vi "Read Multiple Voltage Measurements.vi"(8 "error in (no error)":errorcluster, 10 "Multiple Voltage Measurement Type (0:DC)":u16(ring) items=["Voltage", "Voltage Harmonic Amplitude", "Voltage Harmonic Phase"], 11 "VISA resource name":refnum<visa-resource-name>) -> (0 "error out":errorcluster, 2 "Voltage Measurements":sgl[](array[numeric]), 3 "VISA resource name out":refnum<visa-resource-name>)   [LabVIEW 2013, in "California Instruments iX Series.lvlib"]
doc: "Reads the multiple voltage measurements based on the user selectable measurement type."
uses:
  California Instruments iX Series.lvlib
panel:
  out "size(s)":i32
  out "Serial Settings:Number of Bytes at Serial Port":u32
  out "return count":u32
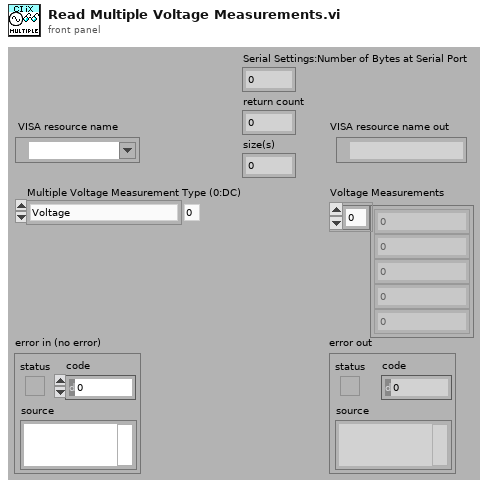
[diagram p1: front panel]
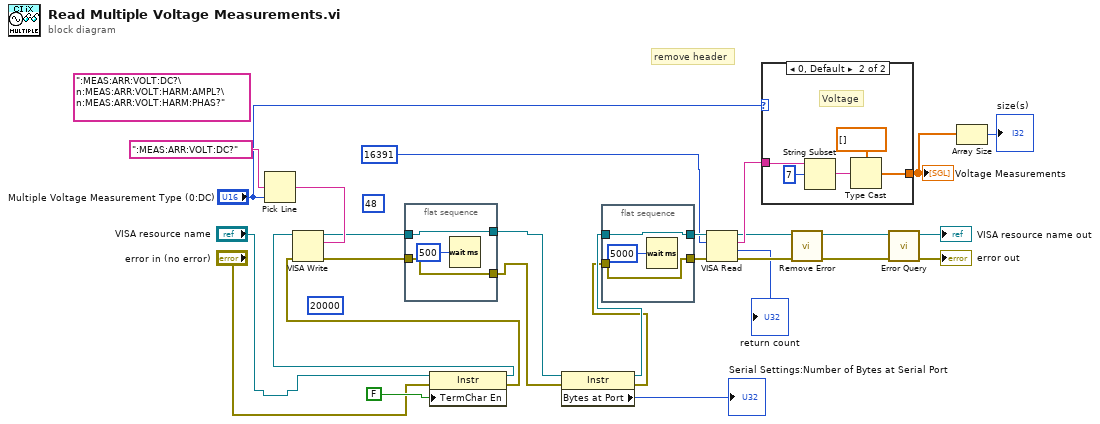
[diagram p0: block diagram]
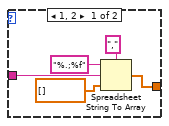
[diagram p2: hidden frame]
diagram:
  (unwired) u16 48 ("mask (16)")
  (unwired) u32 20000 ("size (4096)")
  (unwired) ":MEAS:ARR:VOLT:DC?\n:MEAS:ARR:VOLT:HARM:AMPL?\n:MEAS:ARR:VOLT:HARM:PHAS?" ("multi-line string")
  # "remove header"
  n1 = Pick Line(multi-line string=":MEAS:ARR:VOLT:DC?", line index="Multiple Voltage Measurement Type (0:DC)") -> (output string=w25:string)  [unwired: 1 in]
  n2 = flat-sequence {
    tunnel: w15 -> [w30]
    tunnel: [w30] -> w7
    tunnel: w14 -> [w29]
    tunnel: [w29] -> w6
    frame #0 {
      n3 = Wait (ms)(milliseconds to wait=u32 500) -> ()  [unwired: 1 out]
    }
  }
  n4 = property class="Instr"(reference="VISA resource name", error in="error in (no error)", "TermChar En"=FALSE ("Message Based Settings:Termination Character Enable")) -> (reference out=w9:refnum<visa-resource-name>, error out=w8:errorcluster)
  n5 = VISA Write(VISA resource name=w9, write buffer=w25, error in (no error)=w8) -> (VISA resource name out=w15:refnum<visa-resource-name>, error out=w14:errorcluster)  [unwired: 1 out]
  n6 = property class="Instr"(reference=w7, error in=w6) -> (reference out=w5:refnum<visa-resource-name>, error out=w4:errorcluster, "Bytes at Port"=→"Serial Settings:Number of Bytes at Serial Port":u32)
  n7 = flat-sequence {
    tunnel: w5 -> [w33]
    tunnel: [w33] -> w17
    tunnel: [w32] -> w16
    tunnel: w4 -> [w32]
    frame #0 {
      n8 = Wait (ms)(milliseconds to wait=u32 5000) -> ()  [unwired: 1 out]
    }
  }
  n9 = VISA Read(VISA resource name=w17, byte count=u32 16391, error in (no error)=w16) -> (VISA resource name out=w22:refnum<visa-resource-name>, read buffer=w24:string, return count=→"return count":u32, error out=w21:errorcluster)
  n10 = case shown="0, Default" "Multiple Voltage Measurement Type (0:DC)" {
    tunnel: w24 -> [w39 w44]
    tunnel: [w36 w40] -> w13
    frame 1, 2 {
      n11 = Spreadsheet String To Array(delimiter (Tab)=",", format string="%.;%f", spreadsheet string=w39, array type (2D Dbl)=sgl[] []) -> (array=w36:sgl[])
    }
    frame 0, Default {
      # "Voltage"
      n12 = String Subset(string=w44, offset (0)=7) -> (substring=w42:string)  [unwired: 1 in]
      n13 = Type Cast(type=sgl[] [], x=w42) -> (*(type *) &x=w40:sgl[])
    }
  }
  "Voltage Measurements" <- w13
  n14 = call "Remove Error.vi"("error in (no error)"=w21, "VISA resource name"=w22) -> ("error out"=w19:errorcluster, "VISA resource name out"=w20:refnum<visa-resource-name>)  [unwired: 8 in]
  n15 = call "Error Query.vi"("error in (no error)"=w19, "VISA resource name"=w20) -> ("error out"=→"error out":errorcluster, "VISA resource name out"=→"VISA resource name out":refnum<visa-resource-name>)  [unwired: 6 in, 2 out]
  n16 = Array Size(array=w13) -> (size(s)=→"size(s)":i32)
